vi "Gen Next State based on user input.vi"(4 "Next State IN":string, 6 "Generate Event?":bool, 7 "Idle State":string, 8 "Timer before next step (20s)":dbl=20.0, 9 "Continue To Wait State":string, 10 "VI Refnum":refnum<vi>, 11 "SubPanel in":refnum<vi>) -> (3 "Next State Out":string)   [LabVIEW 2011]
uses:
  timerAction_typdef.ctl
  op_typdef.ctl
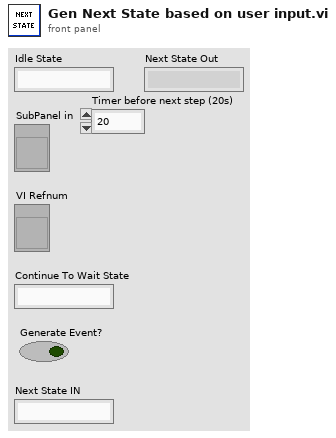
[diagram p1: front panel]
types:
  T1 = typedef "timerAction_typdef.ctl" = enum16{"Idle", "Start Timer", "Timer Running"}
  T2 = typedef "op_typdef.ctl" = enum16{"Idle", "Continue to Wait", "Exit", "Ignore and Continue"}
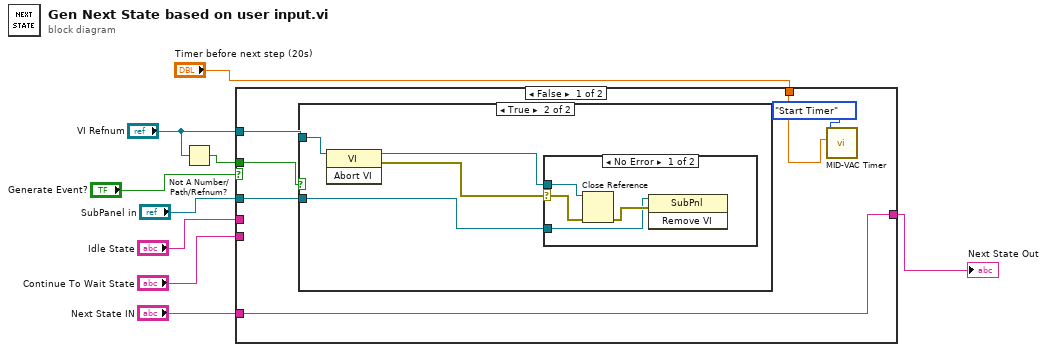
[diagram p0: block diagram]
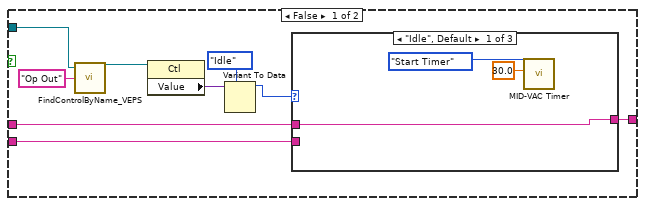
[diagram p5: hidden frame]
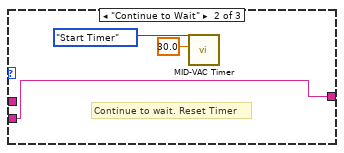
[diagram p6: hidden frame]
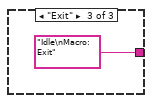
[diagram p7: hidden frame]
diagram:
  n1 = Not A Number/Path/Refnum?(number/path/refnum="VI Refnum") -> (NaN/Path/Refnum?=w9:bool)
  n2 = case shown="False" "Generate Event?" {
    tunnel: [w12 w28] -> w4
    tunnel: w9 -> [w14 w27]
    tunnel: "VI Refnum" -> [w13 w26]
    tunnel: "Next State IN" -> [w12 _]
    tunnel: "Continue To Wait State" -> [_ w25]
    tunnel: "Idle State" -> [_ w24]
    tunnel: "SubPanel in" -> [w11 _]
    tunnel: "Timer before next step (20s)" -> [w10 _]
    frame False {
      n3 = case shown="True" w14 {
        tunnel: w13 -> [_ w19]
        tunnel: w11 -> [_ w16]
        frame False {
        }
        frame True {
          n4 = invoke class="VI" method="Abort VI"(reference=w19) -> (reference out=w17:refnum<vi>, error out=w18:errorcluster)  [unwired: 2 in, 1 out]
          n5 = case shown="No Error" w18 {
            selector: w18 -> [w22 _]
            tunnel: w17 -> [w23 _]
            tunnel: w16 -> [w20 _]
            frame No Error {
              n6 = Close Reference(reference=w23, error in (no error)=w22) -> (error out=w21:errorcluster)
              n7 = invoke on="Invoke Node" class="SubPnl" method="Remove VI"(reference=w20, error in=w21) -> ()  [unwired: 1 in, 3 out]
            }
            frame Error {
            }
          }
        }
      }
      n8 = call "MID-VAC Timer.vi"("TO sec (Start timer)"=w10, "Action"=timerAction_typdef."Start Timer") -> ()  [unwired: 9 in, 1 out]
    }
    frame True {
      # "when to is true\nand"
      n9 = case shown="True" w27 {
        tunnel: [w33 w45] -> w28
        tunnel: w26 -> [w31 _]
        tunnel: w25 -> [w30 w45]
        tunnel: w24 -> [w29 _]
        frame False {
          n10 = call "FindControlByName_VEPS.vi"("control name"="Op Out", "vi refnum"=w31) -> ("control refnum"=w36:refnum<vi>)  [unwired: 2 in, 1 out]
          n11 = property class="Ctl"(reference=w36) -> ("Value"=w35:variant)  [unwired: 1 in, 2 out]
          n12 = Variant To Data(type=op_typdef."Idle" ("Op Out"), Variant=w35) -> (data=w34:T2)  [unwired: 1 in, 1 out]
          n13 = case shown="\"Idle\", Default" w34 {
            tunnel: [w38 w41 "Idle\nMacro: Exit"] -> w33
            tunnel: w30 -> [_ w41 _]
            tunnel: w29 -> [w38 _ _]
            frame "Idle", Default {
              n14 = call "MID-VAC Timer.vi"("TO sec (Start timer)"=30.0, "Action"=timerAction_typdef."Start Timer") -> ()  [unwired: 9 in, 1 out]
            }
            frame "Continue to Wait" {
              # "Continue to wait. Reset Timer"
              n15 = call "MID-VAC Timer.vi"("TO sec (Start timer)"=30.0, "Action"=timerAction_typdef."Start Timer") -> ()  [unwired: 9 in, 1 out]
            }
            frame "Exit" {
            }
          }
        }
        frame True {
        }
      }
    }
  }
  "Next State Out" <- w4
